vi "multiple.vi"(2 "B":T3, 3 "A":T4) -> (0 "Flags":T1, 1 "Result":T2)   [LabVIEW 2013]
panel:
  # "R1"
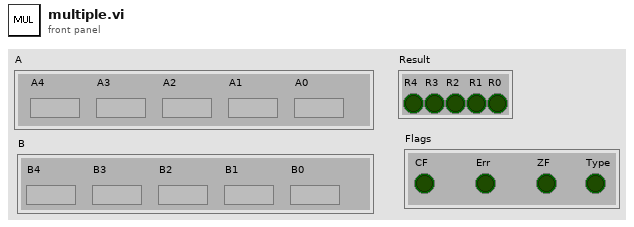
[diagram p1: front panel]
types:
  T1 = cluster{"CF":bool, "Err":bool, "ZF":bool, "Type":bool}
  T2 = cluster{"R4":bool, "R3":bool, "R2":bool, bool, "R0":bool}
  T3 = cluster{"B4":bool, "B3":bool, "B2":bool, "B1":bool, "B0":bool}
  T4 = cluster{"A4":bool, "A3":bool, "A2":bool, "A1":bool, "A0":bool}
  T5 = cluster{"P0":cluster{"X4":bool, "X3":bool, "X2":bool, "X1":bool}, "P1":cluster{"X4":bool, "X3":bool, "X2":bool, "X1":bool, "X0":bool}, "P2":cluster{"X4":bool, "X3":bool, "X2":bool, "X1":bool, "X0":bool}, "P3":cluster{"X4":bool, "X3":bool, "X2":bool, "X1":bool, "X0":bool}, "P4":cluster{"X4":bool, "X3":bool, "X2":bool, "X1":bool, "X0":bool}}
  T6 = cluster{"X4":bool, "X3":bool, "X2":bool, "X1":bool}
  T7 = cluster{"X4":bool, "X3":bool, "X2":bool, "X1":bool, "X0":bool}
  T8 = cluster{bool, "X4":bool, "X3":bool, "X2":bool, "X1":bool}
  T9 = cluster{"Y4":bool, "Y3":bool, "Y2":bool, "Y1":bool, "Y5":bool}
  T10 = cluster{"Y0":bool, "Y0":bool, "Y0":bool, "Y0":bool, "X0":bool}
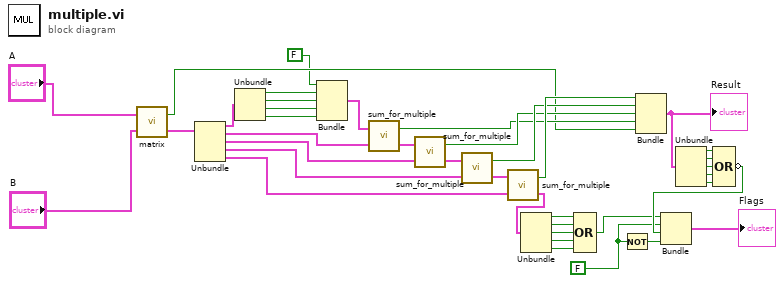
[diagram p0: block diagram]
diagram:
  w1 = FALSE
  n1 = call "matrix.vi"("B"="B", "A"="A") -> ("P"=w37:T5, "X0"=w23:bool)
  n2 = Unbundle(w37) -> ("P0"=w36:T6, "P1"=w34:T7, "P2"=w32:T7, "P3"=w30:T7, "P4"=w28:T7)
  n3 = Unbundle(w36) -> ("X4"=w19:bool, "X3"=w20:bool, "X2"=w21:bool, "X1"=w22:bool)
  n4 = Bundle(FALSE, "X4"=w19, "X3"=w20, "X2"=w21, "X1"=w22) -> (w35:T8)  [unwired: 1 in]
  n5 = call "sum_for_multiple.vi"("B"=w34, "A"=w35) -> ("Output"=w33:T9, "Y0"=w24:bool)
  n6 = call "sum_for_multiple.vi"("B"=w32, "A"=w33) -> ("Output"=w31:T9, "Y0"=w25:bool)
  n7 = call "sum_for_multiple.vi"("B"=w30, "A"=w31) -> ("Output"=w29:T9, "Y0"=w26:bool)
  n8 = call "sum_for_multiple.vi"("B"=w28, "A"=w29) -> ("Output"=w4:T9, "Y0"=w27:bool)
  n9 = Unbundle(w4) -> ("Y4"=w9:bool, "Y3"=w8:bool, "Y2"=w7:bool, "Y1"=w6:bool, "Y5"=w5:bool)
  n10 = Compound Arithmetic op=OR(w9, w8, w7, w6, w5) -> (w3:bool)
  n11 = Not(x=w1) -> (.not. x?=w2:bool)
  n12 = Bundle("Y0"=w27, "Y0"=w26, "Y0"=w25, "Y0"=w24, "X0"=w23) -> (w11:T10)  [unwired: 1 in]
  "Result" <- w11
  n13 = Unbundle(w11) -> ("Y0"=w16:bool, "Y0"=w15:bool, "Y0"=w14:bool, "Y0"=w13:bool, "X0"=w12:bool)
  n14 = Compound Arithmetic op=OR(w16, w15, w14, w13, w12) -> (invert w10:bool)
  n15 = Bundle(w3, w1, w10, w2) -> (→"Flags":cluster{bool, bool, bool, bool})  [unwired: 1 in]
